vi "AutoAim.vi"(8 "error in (no error)":errorcluster) -> (0 "error out":errorcluster)   [LabVIEW 2013]
uses:
  Robot Global Data.vi
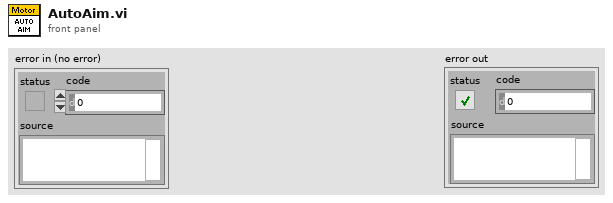
[diagram p1: front panel]
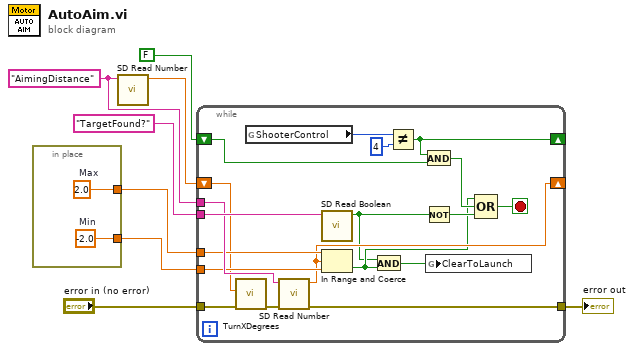
[diagram p0: block diagram]
diagram:
  w6 = "AimingDistance" ("Name")
  n1 = in-place {
    in-place-border: [w10] -> w3
    in-place-border: [w9] -> w2
    w9 = -2.0  # Min
    w10 = 2.0  # Max
  }
  n2 = call <vilib>:"SD Read Number.vi"("Name"=w6) -> ("Numeric"=w5:dbl)  [unwired: 8 in, 2 out]
  n3 = while {
    tunnel: "TargetFound?" ("Name") -> [w29]
    tunnel: w6 -> [w28]
    tunnel: "error in (no error)" -> [w27]
    shift-right: [w15] -> _
    shift-left: w5 -> [w14]
    tunnel: [w19] -> w4
    tunnel: w3 -> [w26]
    tunnel: w2 -> [w25]
    shift-right: [w22] -> _
    shift-left: FALSE -> [w21]
    stop <- w16 stop-if-true
    n4 = call "TurnXDegrees.vi"("error in (no error)"=w27, "degrees"=w14) -> ("error out"=w20:errorcluster)  [unwired: 9 in]
    n5 = global read "Robot Global Data.vi" "ShooterControl"() -> (w24:u32)
    n6 = call <vilib>:"SD Read Number.vi"("error in"=w20, "Name"=w28) -> ("error out"=w19:errorcluster, "Numeric"=w15:dbl)  [unwired: 7 in, 1 out]
    n7 = call <vilib>:"SD Read Boolean.vi"("Name"=w29) -> ("Boolean"=w12:bool)  [unwired: 8 in, 2 out]
    n8 = In Range and Coerce(upper limit=w26, x=w15, lower limit=w25) -> (In Range?=w13:bool)  [unwired: 1 out]
    n9 = And(x=w12, y=w13) -> (x .and. y?=w11:bool)
    n10 = Not Equal?(x=w24, y=u32 4) -> (x != y?=w22:bool)
    n11 = And(x=w22, y=w21) -> (x .and. y?=w18:bool)
    n12 = Not(x=w12) -> (.not. x?=w17:bool)
    n13 = global write "Robot Global Data.vi" "ClearToLaunch"(w11) -> ()
    n14 = Compound Arithmetic op=OR(w13, w18, w17) -> (w16:bool)
  }
  "error out" <- w4
